vi "Close.vi"(2 "Que name":string, 5 "error in":errorcluster) -> (6 "error out":errorcluster)   [LabVIEW 2014, in "Que lib.lvlib"]
uses:
  Que lib.lvlib
  Controls/Queue cluster.ctl
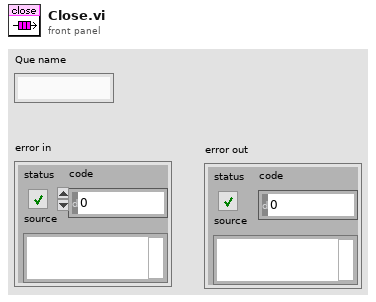
[diagram p1: front panel]
types:
  T1 = typedef "Que lib.lvlib/Queue cluster.ctl" = cluster{"Message":string, "Data":variant}
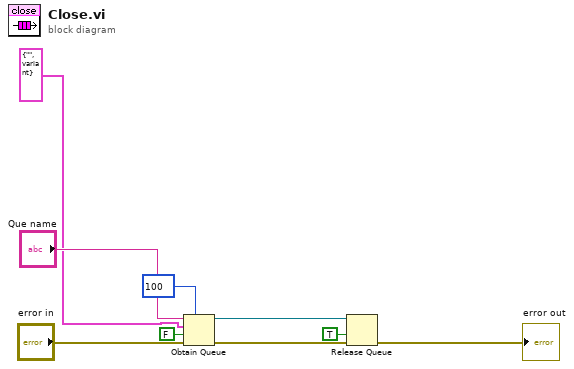
[diagram p0: block diagram]
diagram:
  n1 = Obtain Queue(max queue size (-1, unlimited)=100, name (unnamed)="Que name", element data type=T1 {"Message"="", "Data"=variant} ("Queue Cluster"), create if not found? (T)=FALSE, error in (no error)="error in") -> (queue out=w8:refnum<queue>, error out=w9:errorcluster)  [unwired: 1 out]
  n2 = Release Queue(queue=w8, force destroy? (F)=TRUE, error in (no error)=w9) -> (error out=→"error out":errorcluster)  [unwired: 2 out]
